vi "Signal Composer.vi"() -> ()   [LabVIEW 2023]
uses:
  <vilib>/express/express analysis/Spectral/Block/exnSpectralBlock spectral measurements RMS poly.vi
  <vilib>/express/express analysis/Spectral/Block/exnSpectralBlock spectral measurements RMS DDT.vi
  <vilib>/express/express analysis/Spectral/XNode/ExpressSpectralMeasurementsBlockNode.xnode
panel:
  in  "?":string
  in  "Play Waveform":bool
  in  "?":bool
  in  "High Cutoff":dbl(slide) scale=20.0..20000.0
  in  "Low Cutoff":dbl(slide) scale=20.0..20000.0
  in  "Filter Type":i64(knob) min=0 max=3 step=1 scale=0.0..3.0 scale format="%o"
  out "Waveform":dynamicdata(graph)
  out "Spectrum":dynamicdata(graph)
  in  "?":T1(array[cluster]) {"Wave Type" scale=0.0..3.0; "Amplitude" scale=0.0..10.0; "Frequency" scale=20.0..20000.0}
  # "off"
  # "on"
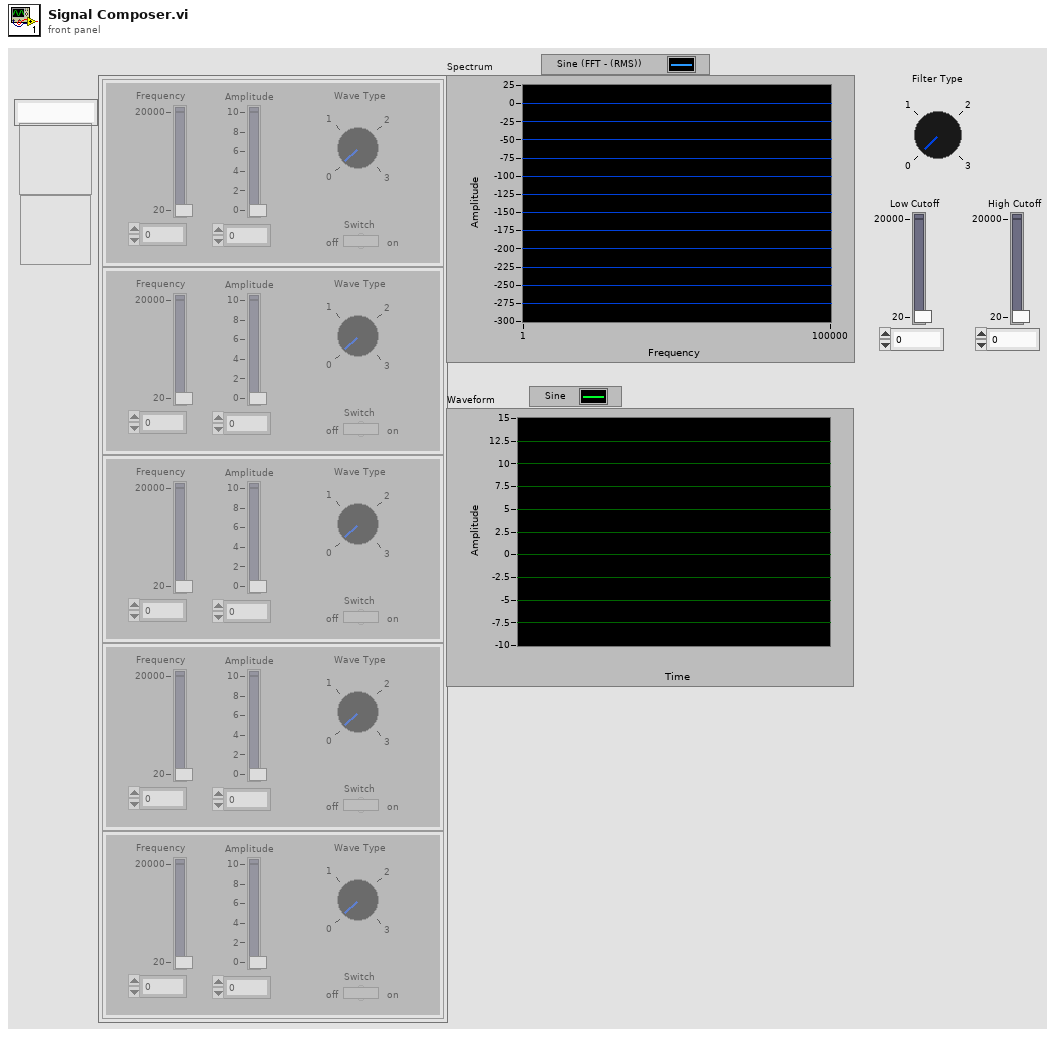
[diagram p1: front panel]
types:
  T1 = cluster{"Frequency":dbl, "Amplitude":dbl, "Wave Type":i64, "Switch":bool}[]
  T2 = cluster{"averaging mode":u16, "weighting mode":u16, "number of averages":u32}
  T3 = cluster{"dB On (F)":bool, "unwrap phase (F)":bool, "convert to degree (F)":bool}
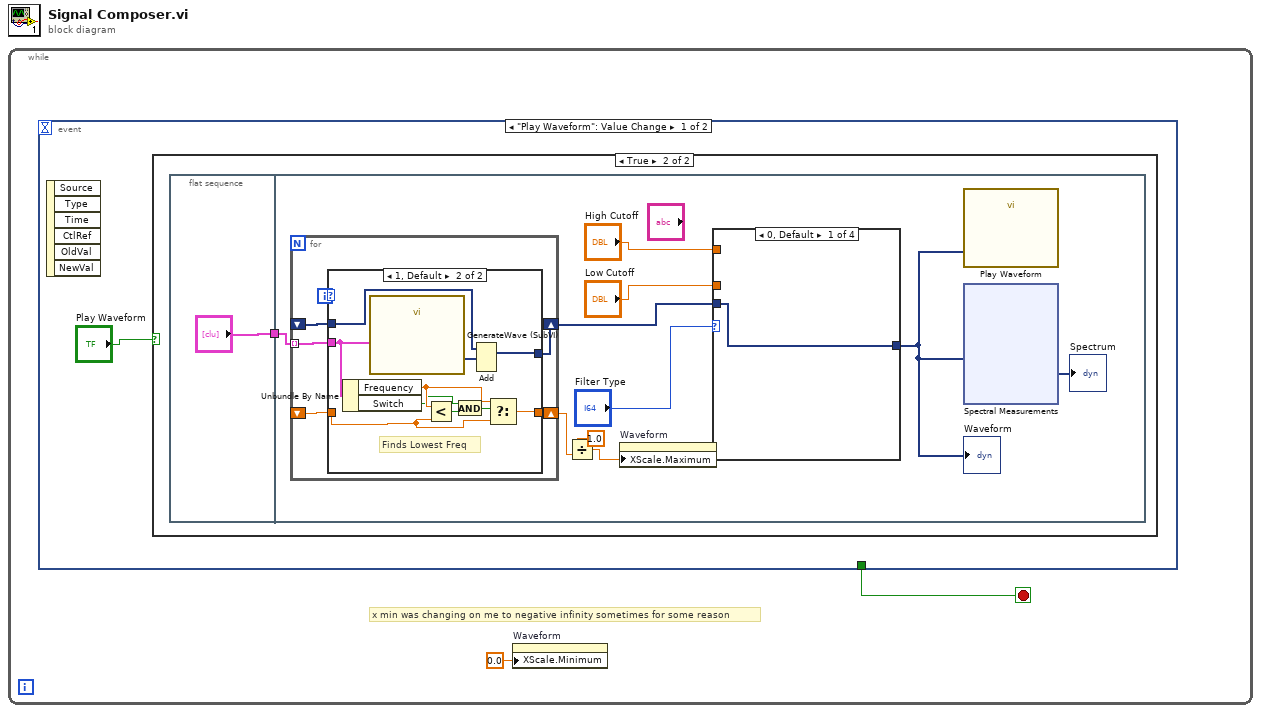
[diagram p0: block diagram]
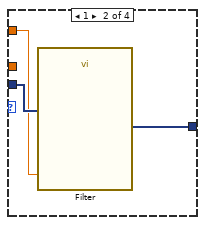
[diagram p3: hidden frame]
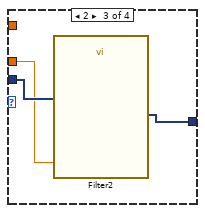
[diagram p4: hidden frame]
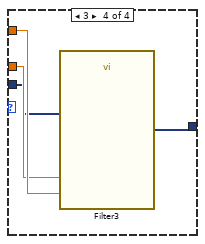
[diagram p5: hidden frame]
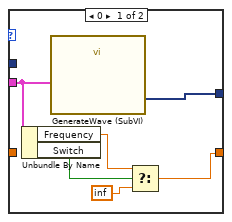
[diagram p6: hidden frame]
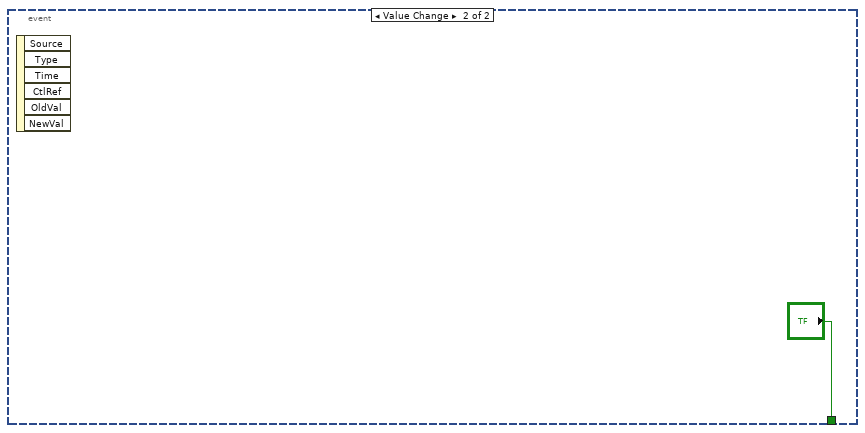
[diagram p7: hidden frame]
diagram:
  n1 = while {
    stop <- w2 stop-if-true
    # "x min was changing on me to negative infinity sometimes for some reason"
    n2 = event shown="[0] \"Play Waveform\": Value Change" {
      selector: _ -> [_ _]
      dyn-events: _ -> [_ _]
      timeout: _ -> [_ _]
      tunnel: [_ "?"] -> w2
      event "Play Waveform": Value Change {
        n3 = event-data() -> ()  [unwired: 1 in, 6 out]
        n4 = case shown="True" "Play Waveform" {
          frame False {
          }
          frame True {
            n5 = flat-sequence {
              tunnel: ["?"] -> w4
              tunnel: w4 -> [w15]
              frame #0 {
              }
              frame #1 {
                n6 = for {
                  tunnel: w15 -> [w41] mode=indexing
                  shift-right: [w39] -> w13
                  shift-left: _ -> [w40]
                  shift-right: [w38] -> w7
                  shift-left: _ -> [w37]
                  i -> [w42]
                  n7 = case shown="1, Default" w42 {
                    tunnel: w41 -> [w47 w54]
                    tunnel: w40 -> [_ w56]
                    tunnel: [w48 w57] -> w39
                    tunnel: [w45 w55] -> w38
                    tunnel: w37 -> [_ w52]
                    frame 0 {
                      n8 = Unbundle By Name(w47) -> ("Frequency"=w44:dbl, "Switch"=w46:bool)
                      n9 = call "GenerateWave (SubVI).vi"("wave"=w47) -> ("DC"=w48:dynamicdata)  [unwired: 10 in]
                      n10 = Select(t=w44, s=w46, f=inf) -> (s? t:f=w45:dbl)
                    }
                    frame 1, Default {
                      # "Finds Lowest Freq"
                      n11 = Unbundle By Name(w54) -> ("Frequency"=w53:dbl, "Switch"=w50:bool)
                      n12 = call "GenerateWave (SubVI).vi"("wave"=w54) -> ("DC"=w58:dynamicdata)  [unwired: 10 in]
                      n13 = Less?(x=w53, y=w52) -> (x < y?=w49:bool)
                      n14 = And(x=w50, y=w49) -> (x .and. y?=w51:bool)
                      n15 = Add(1:w58, 2:w56) -> (0:w57:dynamicdata)  [unwired: 1 in, 1 out]
                      n16 = Select(t=w53, s=w51, f=w52) -> (s? t:f=w55:dbl)
                    }
                  }
                }
                n17 = Divide(x=1.0, y=w7) -> (x/y=w8:dbl)
                n18 = property on="Waveform" class="WFGraph (strict)"("XScale.Maximum"=w8) -> ()  [unwired: 2 in, 2 out]
                n19 = case shown="0, Default" "Filter Type" {
                  tunnel: w13 -> [w16 w19 w21 w23]
                  tunnel: [w16 w18 w22 w24] -> w12
                  tunnel: "High Cutoff" -> [_ w17 _ w26]
                  tunnel: "Low Cutoff" -> [_ _ w20 w25]
                  frame 0, Default {
                  }
                  frame 1 {
                    n20 = call "Filter"("Lower Cut-Off"=w17, "Signal"=w19) -> ("Filtered Signal"=w18:dynamicdata)  [unwired: 8 in, 1 out]
                  }
                  frame 2 {
                    n21 = call "Filter2"("Lower Cut-Off"=w20, "Signal"=w21) -> ("Filtered Signal"=w22:dynamicdata)  [unwired: 8 in, 1 out]
                  }
                  frame 3 {
                    n22 = call "Filter3"("Lower Cut-Off"=w25, "Upper Cut-Off"=w26, "Signal"=w23) -> ("Filtered Signal"=w24:dynamicdata)  [unwired: 7 in, 1 out]
                  }
                }
                "Waveform" <- w12
                n23 = call "Play Waveform"("Data"=w12) -> ()  [unwired: 18 in, 1 out]
                n24 = xnode "Spectral Measurements"("Signals"=w12) -> ("FFT - (RMS)"=→"Spectrum":dynamicdata)  [unwired: 1 in, 2 out]
              }
            }
          }
        }
      }
      event Value Change {
        n25 = event-data() -> ()  [unwired: 1 in, 6 out]
      }
    }
    n26 = property on="Waveform" class="WFGraph (strict)"("XScale.Minimum"=0.0 ("X Scale.Range:Minimum")) -> ()  [unwired: 2 in, 2 out]
  }
